vi "MatrixToData5.vi"(7 "database variant":variant, 8 "database variant 5":variant, 9 "database variant 4":variant, 10 "database variant 3":variant, 11 "database variant 2":variant) -> (0 "data 5":string, 1 "data 4":string, 2 "data 3":string, 3 "data 2":string, 5 "data":string)   [LabVIEW 2012]
uses:
  <vilib>/addons/database/_DB Variant To Data/Database Variant To Data.xnode
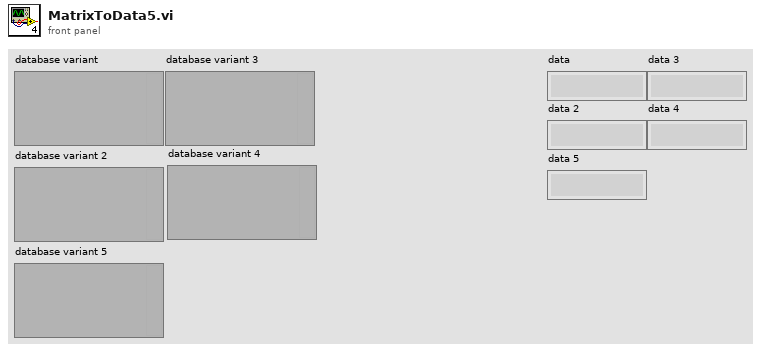
[diagram p1: front panel]
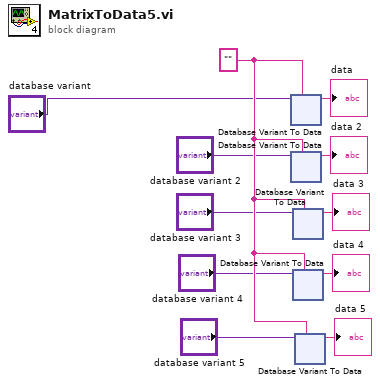
[diagram p0: block diagram]
diagram:
  w11 = ""
  n1 = xnode "Database Variant To Data"("database variant"="database variant", "type"=w11) -> ("data"=→"data":string)  [unwired: 1 in, 1 out]
  n2 = xnode "Database Variant To Data"("database variant"="database variant 2", "type"=w11) -> ("data"=→"data 2":string)  [unwired: 1 in, 1 out]
  n3 = xnode "Database Variant To Data"("database variant"="database variant 3", "type"=w11) -> ("data"=→"data 3":string)  [unwired: 1 in, 1 out]
  n4 = xnode "Database Variant To Data"("database variant"="database variant 4", "type"=w11) -> ("data"=→"data 4":string)  [unwired: 1 in, 1 out]
  n5 = xnode "Database Variant To Data"("database variant"="database variant 5", "type"=w11) -> ("data"=→"data 5":string)  [unwired: 1 in, 1 out]
